vi "LinInterp_PercdentFlow to uA.vi"(10 "Target":dbl=28.0) -> (2 "uA Output":i32)   [LabVIEW 2009]
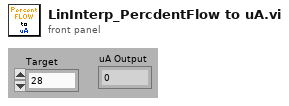
[diagram p1: front panel]
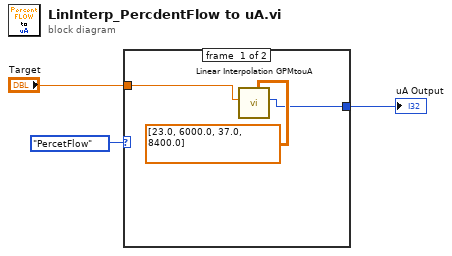
[diagram p0: block diagram]
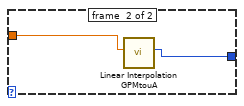
[diagram p2: hidden frame]
diagram:
  n1 = case shown="\"PercetFlow\", Default" enum16{"GPM", "PercetFlow"}."PercetFlow" ("Enum") {
    tunnel: "Target" -> [w5 w8]
    tunnel: [w4 w7] -> w2
    frame #0 {
      n2 = call "Linear Interpolation GPMtouA.vi"("2D Flow Data (GPM,uA)"=dbl[][] [[23.0, 6000.0], [37.0, 8400.0]] ("Interpolation Table(Xs,Ys)"), "GPM Target"=w5) -> ("uA Output"=w4:i32)  [unwired: 9 in]
    }
    frame #1 {
      n3 = call "Linear Interpolation GPMtouA.vi"("GPM Target"=w8) -> ("uA Output"=w7:i32)  [unwired: 10 in]
    }
  }
  "uA Output" <- w2
